vi "ReadbyRefBool.vi"(8 "error in":errorcluster caption="entrée d'erreur", 11 "Control Ref":refnum<vi>) -> (0 "error out":errorcluster caption="sortie d'erreur", 3 "Valeur":bool)   [LabVIEW 2019]
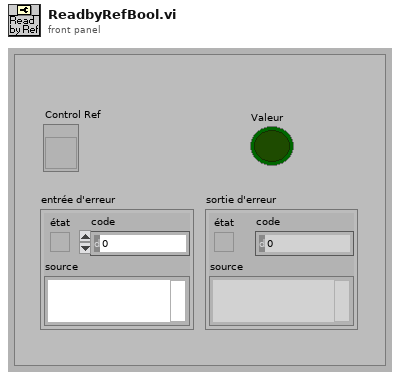
[diagram p1: front panel]
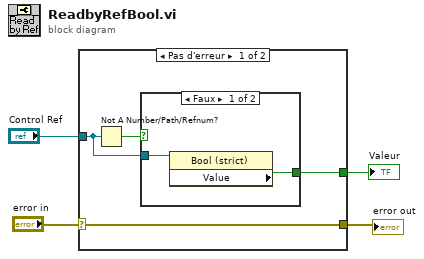
[diagram p0: block diagram]
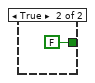
[diagram p2: hidden frame]
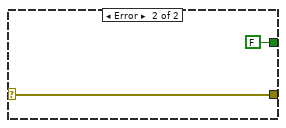
[diagram p3: hidden frame]
diagram:
  n1 = case shown="Pas d'erreur" "error in" {
    selector: "error in" -> [w5 w13]
    tunnel: "Control Ref" -> [w7 _]
    tunnel: [w6 FALSE ("Value")] -> w3
    tunnel: [w5 w13] -> w1
    frame No Error {
      n2 = Not A Number/Path/Refnum?(number/path/refnum=w7) -> (NaN/Path/Refnum?=w8:bool)
      n3 = case shown="Faux" w8 {
        tunnel: w7 -> [w10 _]
        tunnel: [w9 FALSE ("Value")] -> w6
        frame False {
          n4 = property class="Bool (strict)"(reference=w10) -> ("Value"=w9:bool)  [unwired: 1 in, 2 out]
        }
        frame True {
        }
      }
    }
    frame Error {
    }
  }
  "Valeur" <- w3
  "error out" <- w1
